vi "Day04-01_변수2 (글로벌 변수).vi"() -> ()   [LabVIEW 2021]
panel:
  in  "불리언 3":bool
  in  "불리언 2":bool
  out "숫자형 2":dbl
  in  "문자열":string
  in  "불리언":bool
  in  "숫자형":dbl
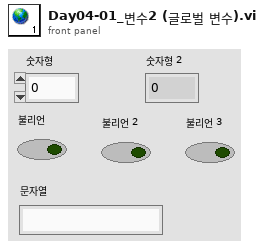
[diagram p1: front panel]
diagram:
